vi "v1.vi"() -> ()   [LabVIEW 2012]
uses:
  <vilib>/measure/NI_MABase.lvlib
  <vilib>/ptbypt/NI_PtbyPt.lvlib
panel:
  out "mean":dbl format="%0.2f"
  out "Waveform Graph 3":waveform(dbl)(graph)
  out "Waveform Graph 2":waveform(dbl)(graph)
  in  "standard deviation":dbl=1.0 format="%.2p"
  out "Y min":dbl format="%0.2f"
  out "Y max":dbl format="%0.2f"
  in  "phase":dbl format="%.2p"
  out "Waveform Graph":waveform(dbl)(graph)
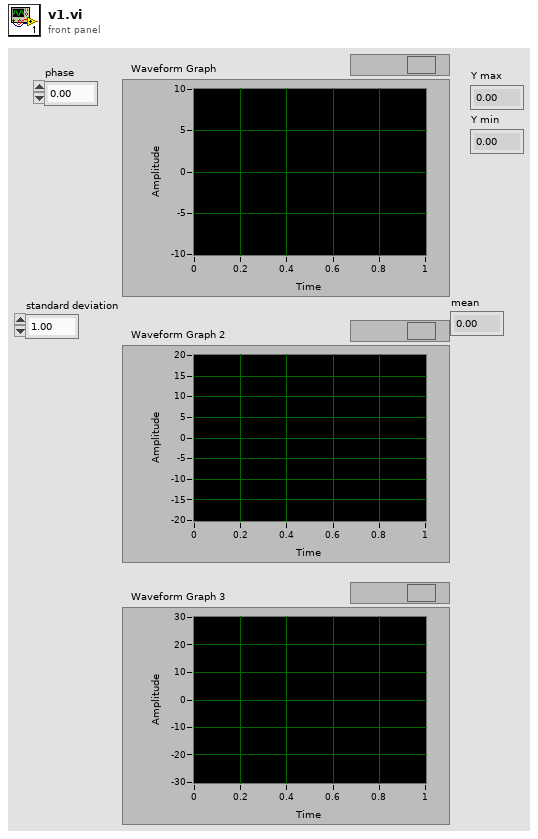
[diagram p1: front panel]
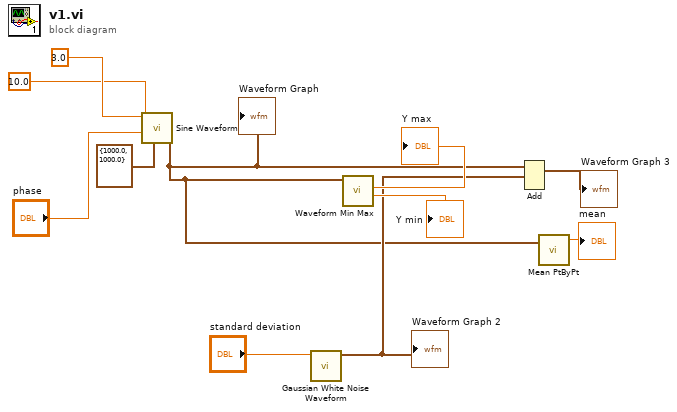
[diagram p0: block diagram]
diagram:
  n1 = call <vilib>:"Sine Waveform.vi"("sampling info"=cluster{"Fs":dbl, "#s":dbl} {"Fs"=1000.0, "#s"=1000.0}, "phase"="phase", "amplitude"=10.0, "frequency"=3.0) -> ("signal out"=w2:waveform(dbl))  [unwired: 6 in, 1 out]
  "Waveform Graph" <- w2
  n2 = call <vilib>:"Gaussian White Noise Waveform.vi"("standard deviation"="standard deviation") -> ("signal out"=w4:waveform(dbl))  [unwired: 9 in, 1 out]
  "Waveform Graph 2" <- w4
  n3 = call <vilib>:"Waveform Min Max.vi"("waveform in"=w2) -> ("Y min"=→"Y min":dbl, "Y max"=→"Y max":dbl)  [unwired: 5 in, 4 out]
  n4 = Add(1:w4, 2:w2) -> (0:→"Waveform Graph 3":waveform(dbl))  [unwired: 1 in, 1 out]
  n5 = call <vilib>:"Mean PtByPt.vi"("x"=w2) -> ("mean"=→"mean":dbl)  [unwired: 3 in, 1 out]
